vi "Connection Monitor - Stop.vi"(8 "error in (no error)":errorcluster, 11 "RemoteControl.STM in":refnum<class "RemoteControl.STM.lvclass">) -> (0 "error out":errorcluster, 3 "RemoteControl.STM out":refnum<class "RemoteControl.STM.lvclass">)   [LabVIEW 2019, in "RemoteControl.STM.lvclass"]
uses:
  RemoteControl.STM.lvclass
  RemoteControl.STM.lvclass/RemoteControl.STM.ctl
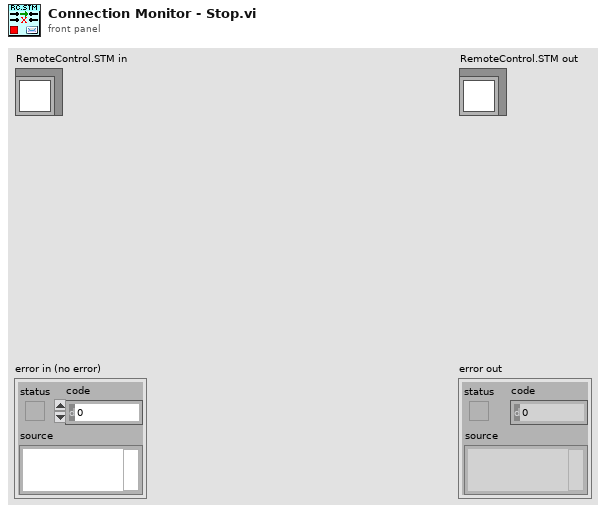
[diagram p1: front panel]
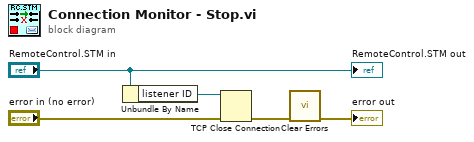
[diagram p0: block diagram]
diagram:
  n1 = Unbundle By Name("RemoteControl.STM in") -> ("listener ID"=w4:refnum<k5>)
  n2 = TCP Close Connection(connection ID=w4, error in (no error)="error in (no error)") -> (error out=w2:errorcluster)  [unwired: 1 in, 1 out]
  n3 = call <vilib>:"Clear Errors.vi"("error in (no error)"=w2) -> ("error out"=→"error out":errorcluster)  [unwired: 5 in, 1 out]
  "RemoteControl.STM out" <- "RemoteControl.STM in"
